vi "Main.vi"() -> ()   [LabVIEW 2015]
uses:
  controls/SwitchStates.ctl
  controls/RT-Variables.lvlib
panel:
  out "FTT Array Temperature":i32
  out "Image":T1(plugin-control)
  out "FEM Temperature":dbl[](array[numeric])
  out "FTT Comm.":bool
  in  "calMirrorSim":bool caption="Cal. Mirror"
  out "RemoteState":T2
  in  "envCoverSim":bool caption="Env. Cover"
  in  "stop comm":bool
  # "Status"
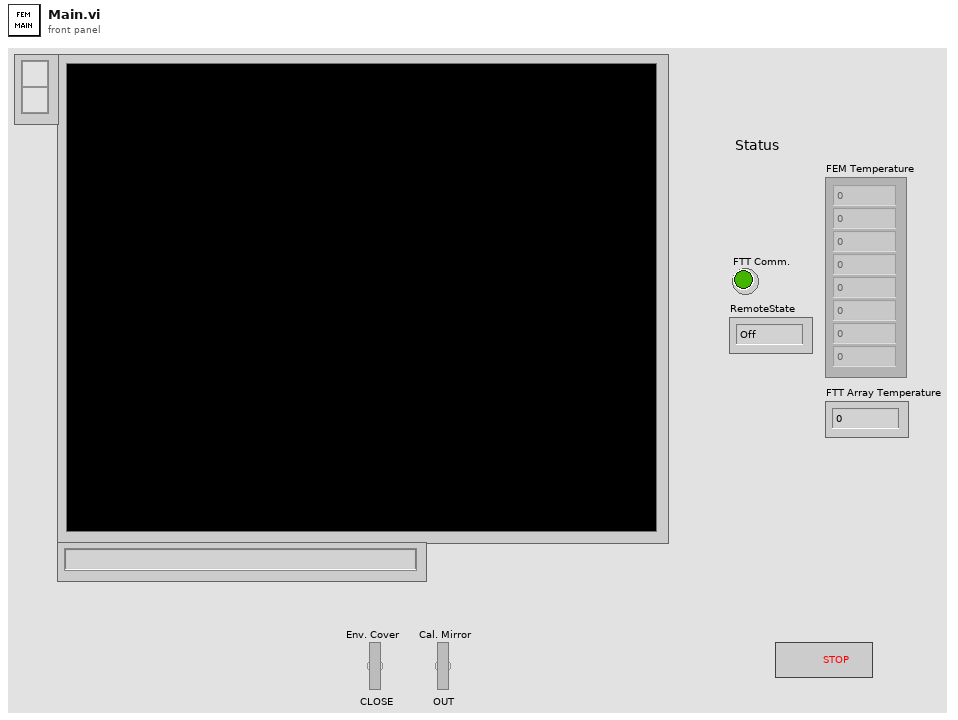
[diagram p1: front panel]
types:
  T1 = typedef "IMAQ Image.ctl" = refnum<image>
  T2 = typedef "RT-Variables.lvlib/SwitchStates.ctl" = enum16{"Off", "Local", "Remote"}
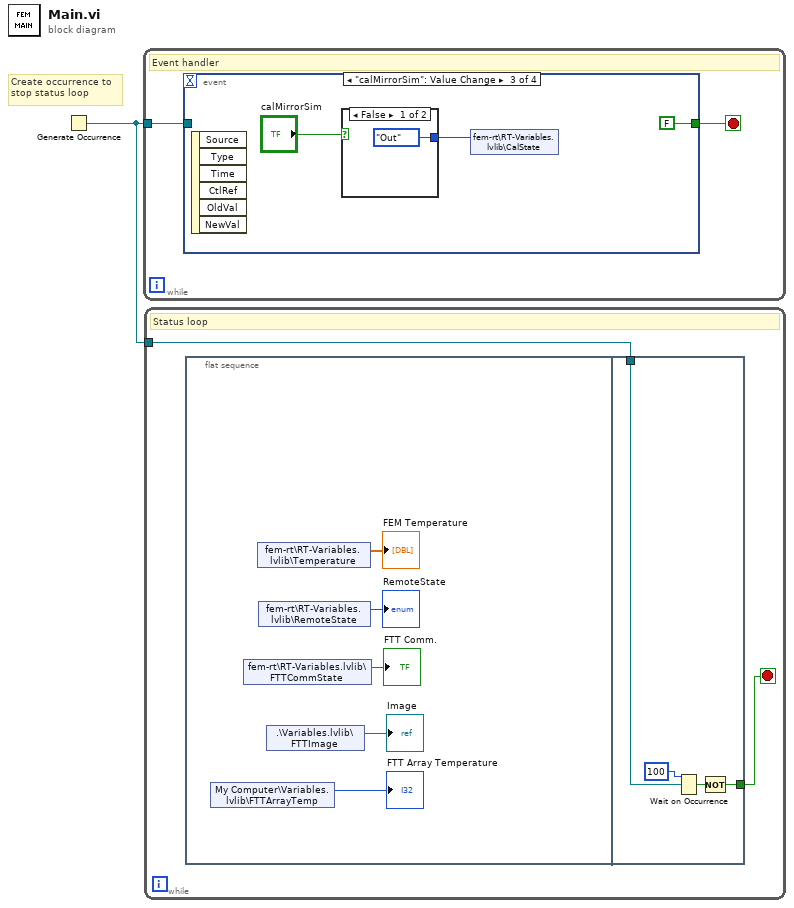
[diagram p0: block diagram]
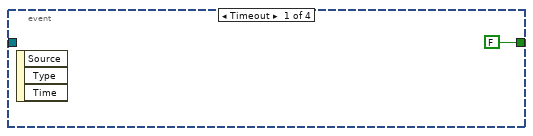
[diagram p2: hidden frame]
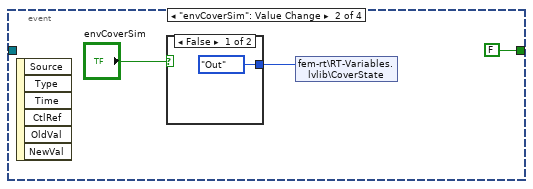
[diagram p3: hidden frame]
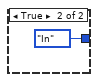
[diagram p4: hidden frame]
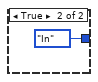
[diagram p5: hidden frame]
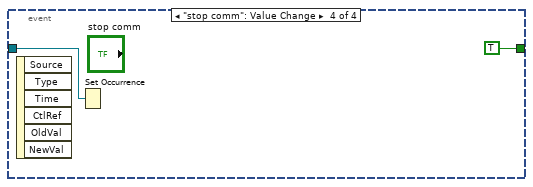
[diagram p6: hidden frame]
diagram:
  # "Create occurrence to\nstop status loop"
  n1 = Generate Occurrence ("Stop Occurrence")() -> (w1:refnum<k4>)
  n2 = while {
    tunnel: w1 -> [w2]
    stop <- w3 stop-if-true
    # "Event handler"
    n3 = event shown="[2] \"calMirrorSim\": Value Change" {
      selector: _ -> [_ _ _ _]
      dyn-events: _ -> [_ _ _ _]
      timeout: _ -> [_ _ _ _]
      tunnel: [FALSE FALSE FALSE TRUE] -> w3
      tunnel: w2 -> [_ _ _ w15]
      event Timeout {
        n4 = event-data() -> ()  [unwired: 1 in, 3 out]
      }
      event "envCoverSim": Value Change {
        n5 = event-data() -> ()  [unwired: 1 in, 6 out]
        n6 = case shown="False" "envCoverSim" {
          tunnel: [enum16{"In", "Moving", "Out", "Wait"}."Out" ("CoverState") enum16{"In", "Moving", "Out", "Wait"}."In" ("CoverState")] -> w6
          frame False {
          }
          frame True {
          }
        }
        n7 = shared-variable "fem-rt\\RT-Variables.lvlib\\CoverState"(w6) -> ()  [unwired: 1 in, 1 out]
      }
      event "calMirrorSim": Value Change {
        n8 = event-data() -> ()  [unwired: 1 in, 6 out]
        n9 = case shown="False" "calMirrorSim" {
          tunnel: [enum16{"In", "Moving", "Out", "Wait"}."Out" ("CoverState") enum16{"In", "Moving", "Out", "Wait"}."In" ("CoverState")] -> w11
          frame False {
          }
          frame True {
          }
        }
        n10 = shared-variable "fem-rt\\RT-Variables.lvlib\\CalState"(w11) -> ()  [unwired: 1 in, 1 out]
      }
      event "stop comm": Value Change {
        n11 = event-data() -> ()  [unwired: 1 in, 6 out]
        n12 = Set Occurrence(w15) -> ()
      }
    }
  }
  n13 = while {
    tunnel: w1 -> [w18]
    stop <- w17 stop-if-true
    # "Status loop"
    n14 = flat-sequence {
      tunnel: w18 -> [w27]
      tunnel: [w24] -> w17
      frame #0 {
        n15 = shared-variable "My Computer\\Variables.lvlib\\FTTArrayTemp"() -> (→"FTT Array Temperature":i32)  [unwired: 1 in, 1 out]
        n16 = shared-variable "fem-rt\\RT-Variables.lvlib\\FTTCommState"() -> (→"FTT Comm.":bool)  [unwired: 1 in, 1 out]
        n17 = shared-variable "fem-rt\\RT-Variables.lvlib\\Temperature"() -> (→"FEM Temperature":dbl[])  [unwired: 1 in, 1 out]
        n18 = shared-variable "fem-rt\\RT-Variables.lvlib\\RemoteState"() -> (→"RemoteState":T2)  [unwired: 1 in, 1 out]
        n19 = shared-variable ".\\Variables.lvlib\\FTTImage"() -> (→"Image":refnum<image>)  [unwired: 1 in, 1 out]
      }
      frame #1 {
        n20 = Wait on Occurrence(2:w27, 3:100 ("ms timeout (-1)")) -> (0:w25:bool)  [unwired: 1 in]
        n21 = Not(x=w25) -> (.not. x?=w24:bool)
      }
    }
  }
